vi "Update Inventory.vi"(8 "error in (no error)":errorcluster, 10 "Producto del inventario":i32, 11 "Coffee Actor in":refnum<class "Coffee Actor.lvclass">) -> (0 "error out":errorcluster, 3 "Coffee Actor out":refnum<class "Coffee Actor.lvclass">)   [LabVIEW 2020, in "Coffee Actor.lvlib" / "Coffee Actor.lvclass"]
uses:
  Coffee Actor.lvclass
  Coffee Actor.lvclass/Coffee Actor.ctl
  <vilib>/Utility/config.llb/Read Key (Double).vi
  <vilib>/Utility/config.llb/Write Key (String).vi
  <vilib>/Utility/config.llb/Read Key (String).vi
  <vilib>/Utility/config.llb/NI_LVConfig.lvlib
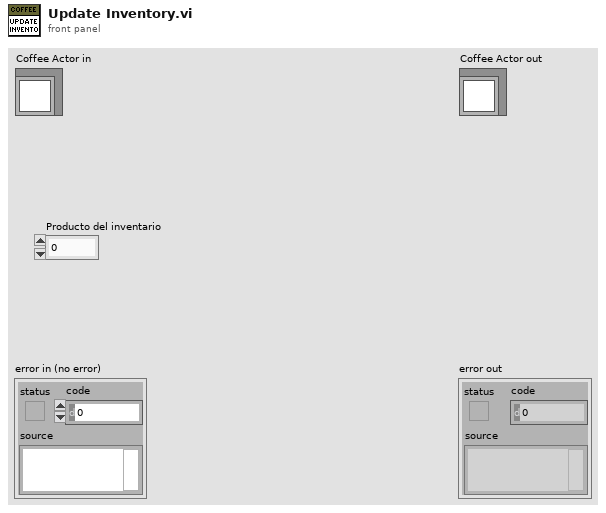
[diagram p1: front panel]
types:
  T1 = typedef "NI_LVConfig.lvlib/Config Data RefNum.ctl" = refnum<k1>
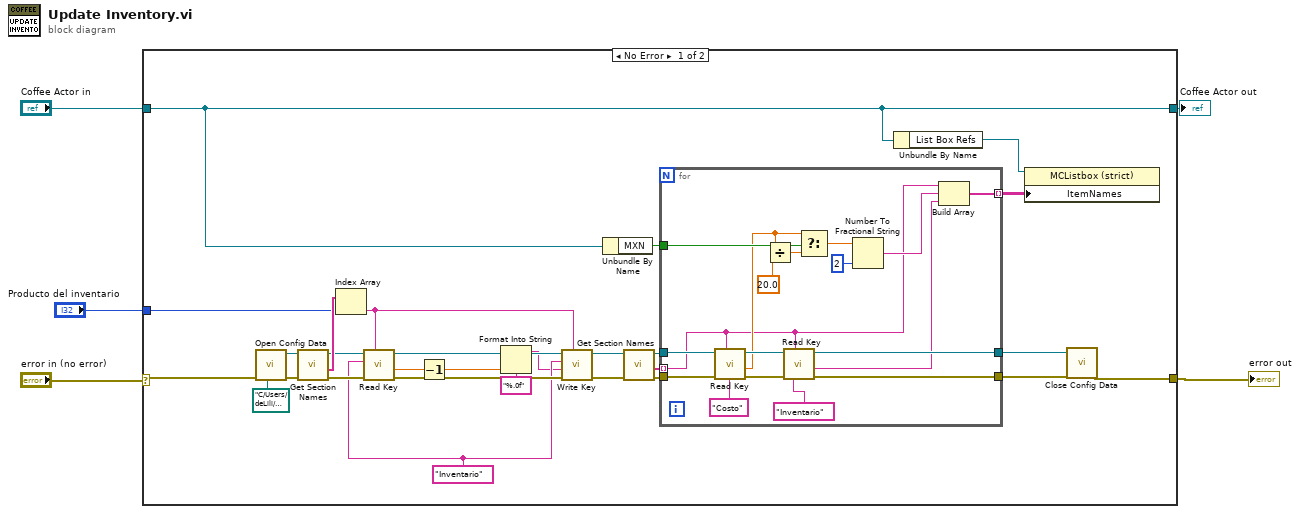
[diagram p0: block diagram]
diagram:
  n1 = case shown="No Error" "error in (no error)" {
    selector: "error in (no error)" -> [w12 w53]
    tunnel: [w7 w53] -> w4
    tunnel: [w11 w52] -> w2
    tunnel: "Coffee Actor in" -> [w11 w52]
    tunnel: "Producto del inventario" -> [w9 _]
    frame No Error {
      w24 = "Inventario" ("key")
      n2 = call <vilib>:"Open Config Data.vi"("error in (no error)"=w12, "configuration file path"=path "C:/Users/deLili/Desktop/UDLSB IET/701/Instrumentacion Virtual/Fork/Maquina-2do-parcial/Coffee Actor.ini") -> ("error out"=w31:errorcluster, "refnum"=w30:T1)  [unwired: 7 in, 1 out]
      n3 = call <vilib>:"Get Section Names.vi"("error in (no error)"=w31, "refnum"=w30) -> ("error out"=w28:errorcluster, "section names"=w29:string[], "refnum out"=w22:T1)  [unwired: 7 in]
      n4 = Index Array(array=w29, index=w9) -> (element=w21:string)
      n5 = call-poly <vilib>:"Read Key.vi"("section"=w21, "error in (no error)"=w28, "key"=w24, "refnum"=w22) -> ("error out"=w26:errorcluster, "value"=w25:dbl, "refnum out"=w23:T1)  [unwired: 4 in, 1 out]
      n6 = Decrement(x=w25) -> (x-1=w19:dbl)
      n7 = Format Into String(format string="%.0f", w19) -> (resulting string=w17:string)  [unwired: 2 in, 1 out]
      n8 = call-poly <vilib>:"Write Key.vi"("section"=w21, "error in (no error)"=w26, "value"=w17, "key"=w24, "refnum"=w23) -> ("error out"=w20:errorcluster, "refnum out"=w16:T1)  [unwired: 4 in, 1 out]
      n9 = Unbundle By Name(w11) -> ("MXN"=w10:bool)
      n10 = call <vilib>:"Get Section Names.vi"("error in (no error)"=w20, "refnum"=w16) -> ("error out"=w15:errorcluster, "section names"=w14:string[], "refnum out"=w13:T1)  [unwired: 7 in]
      n11 = for {
        tunnel: w13 -> [w49]
        tunnel: [w45] -> w6
        tunnel: w15 -> [w51]
        tunnel: [w47] -> w8
        tunnel: w14 -> [w34] mode=indexing
        tunnel: w10 -> [w41]
        tunnel: [w43] -> w33 mode=indexing
        n12 = call-poly <vilib>:"Read Key.vi"("section"=w34, "error in (no error)"=w51, "key"="Costo", "refnum"=w49) -> ("error out"=w50:errorcluster, "value"=w39:dbl, "refnum out"=w46:T1)  [unwired: 4 in, 1 out]
        n13 = Divide(x=w39, y=20.0) -> (x/y=w40:dbl)
        n14 = call-poly <vilib>:"Read Key.vi"("section"=w34, "error in (no error)"=w50, "key"="Inventario", "refnum"=w46) -> ("error out"=w47:errorcluster, "value"=w42:string, "refnum out"=w45:T1)  [unwired: 4 in, 1 out]
        n15 = Select(t=w39, s=w41, f=w40) -> (s? t:f=w37:dbl)
        n16 = Number To Fractional String(number=w37, precision (6)=i16 2) -> (F-format string=w35:string)  [unwired: 2 in]
        n17 = Build Array(w34, w35, w42) -> (w43:string[])
      }
      n18 = Unbundle By Name(w11) -> ("List Box Refs"=w32:refnum<vi>)
      n19 = property class="MCListbox (strict)"(reference=w32, "ItemNames"=w33) -> ()  [unwired: 1 in, 2 out]
      n20 = call <vilib>:"Close Config Data.vi"("error in (no error)"=w8, "refnum"=w6) -> ("error out"=w7:errorcluster)  [unwired: 8 in, 1 out]
    }
    frame Error {
    }
  }
  "error out" <- w4
  "Coffee Actor out" <- w2
